vi "IncStepsMMAvg.vi"(0 "I/O chan for motor pulse":i32=7, 1 "wait time between scans (ms)":i32, 3 "Avg Num":i32=1, 5 "number of scans":i32=128, 9 "Axis":i32=1 min=1 max=4, 11 "Steps to move":i32=100, 13 "Crate File Names":string[](array[string]), 14 "Reverse ?":bool) -> ()   [LabVIEW 2022 SP3]
uses:
  <instrlib>/Acqiris Dx/Acqiris Dx.lvlib
  -MotionRoutines/MotionGlobals.vi
  <vilib>/Analysis/NI_AALBase.lvlib
  <vilib>/Analysis/baseanly.llb/Mean (DBL).vi
panel:
  out "Motion error":bool
  in  "Acq error in":errorcluster
  in  "Board ID":T1=1 min=1 max=32 step=1
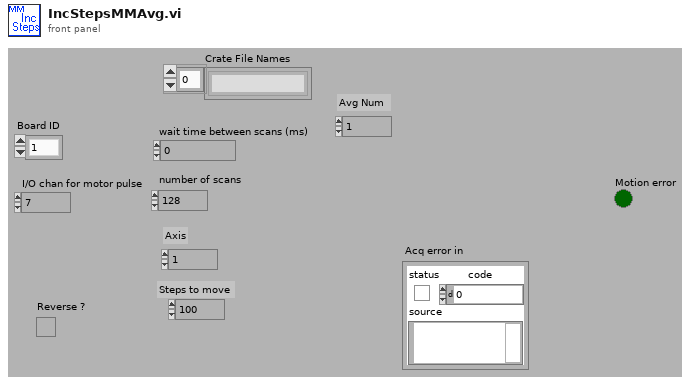
[diagram p1: front panel]
types:
  T1 = typedef "Board Id" = u8
  T2 = cluster{sgl, "Gain [dB]  ":sgl, "Atten (dB)":sgl}[]
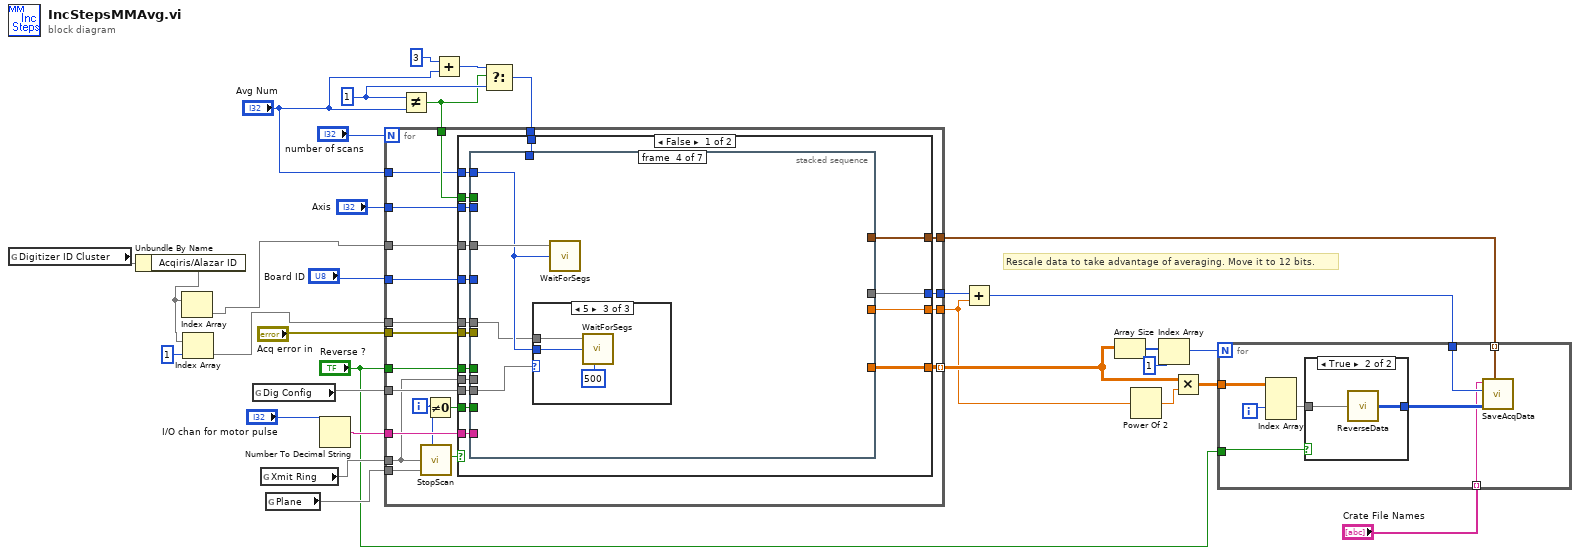
[diagram p0: block diagram]
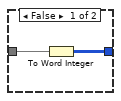
[diagram p2: hidden frame]
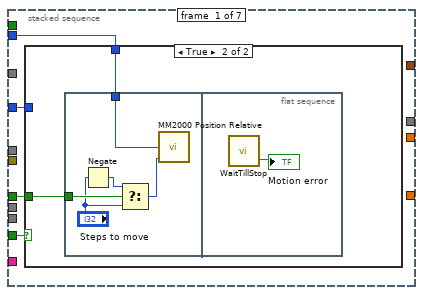
[diagram p3: hidden frame]
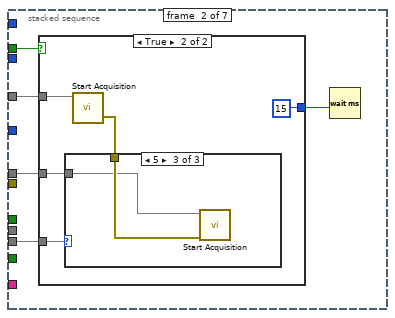
[diagram p5: hidden frame]
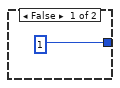
[diagram p6: hidden frame]
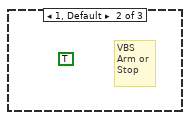
[diagram p8: hidden frame]
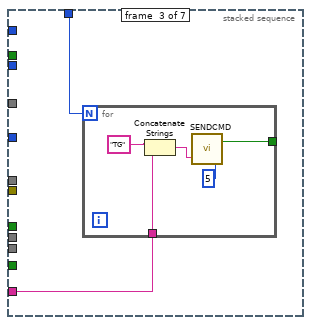
[diagram p9: hidden frame]
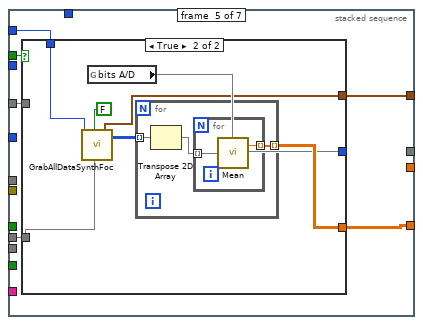
[diagram p12: hidden frame]
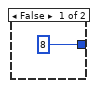
[diagram p13: hidden frame]
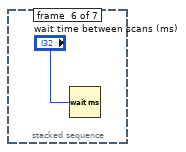
[diagram p14: hidden frame]
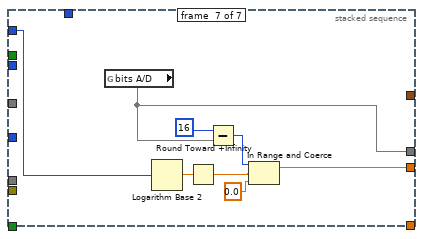
[diagram p15: hidden frame]
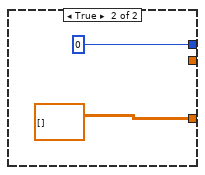
[diagram p16: hidden frame]
diagram:
  w26 = 1
  # "Rescale data to take advantage of averaging. Move it to 12 bits."
  n1 = global read "MotionGlobals.vi" "Digitizer ID Cluster"() -> (w5)
  n2 = Unbundle By Name(w5) -> ("Acqiris/Alazar ID"=w3)
  n3 = Index Array(array=w3) -> (element=w2)  [unwired: 1 in]
  n4 = Index Array(array=w3, index=1) -> (element=w1)
  n5 = global read "MotionGlobals.vi" "Dig Config"() -> (w28)
  n6 = global read "MotionGlobals.vi" "Xmit Ring"() -> (w18)
  n7 = global read "MotionGlobals.vi" "Plane"() -> (w19)
  n8 = Number To Decimal String(number="I/O chan for motor pulse") -> (decimal integer string=w21:string)  [unwired: 1 out]
  n9 = Not Equal?(x=w26, y="Avg Num") -> (x != y?=w23:bool)
  n10 = Add(x=3, y="Avg Num") -> (x+y=w24:i32)
  n11 = Select(t=w24, s=w23, f=w26) -> (s? t:f=w27:i32)
  n12 = for {
    N: "number of scans" -> [_]
    tunnel: "Board ID" -> [w52]
    tunnel: "Axis" -> [w51]
    tunnel: "Reverse ?" -> [w50]
    tunnel: w27 -> [w49]
    tunnel: w2 -> [w48]
    tunnel: "Acq error in" -> [w47]
    tunnel: w28 -> [w46]
    tunnel: [w42] -> w12 mode=indexing
    tunnel: w23 -> [w45]
    tunnel: [w43] -> w8
    tunnel: w21 -> [w40]
    tunnel: "Avg Num" -> [w39]
    tunnel: w19 -> [w37]
    tunnel: w18 -> [w36]
    tunnel: [w35] -> w9
    tunnel: [w34] -> w6
    tunnel: w1 -> [w33]
    i -> [w38]
    n13 = call "StopScan.vi"("Ring"=w36, "Current Plane"=w37, "Line Number"=w38) -> ("Stop Now? Dup"=w41:bool)  [unwired: 1 in, 2 out]
    n14 = Not Equal To 0?(x=w38) -> (x != 0?=w44:bool)
    n15 = case shown="False" w41 {
      tunnel: w52 -> [w69 _]
      tunnel: w51 -> [w68 _]
      tunnel: w50 -> [w67 _]
      tunnel: w49 -> [w66 _]
      tunnel: w48 -> [w65 _]
      tunnel: w47 -> [w64 _]
      tunnel: w46 -> [w63 _]
      tunnel: w45 -> [w62 _]
      tunnel: w44 -> [w61 _]
      tunnel: [w54 u16 0] -> w43
      tunnel: [w60 dbl[][] [] ("Data")] -> w42
      tunnel: w40 -> [w59 _]
      tunnel: w39 -> [w58 _]
      tunnel: w36 -> [w57 _]
      tunnel: [w56 _] -> w35
      tunnel: [w55 _] -> w34
      tunnel: w33 -> [w53 _]
      frame False {
        n16 = stacked-sequence {
          tunnel: w69 -> [w73 _ _ _ _ _ _]
          tunnel: w68 -> [w72 _ _ _ _ _ _]
          tunnel: w67 -> [w71 _ _ _ _ _ _]
          tunnel: w66 -> [_ _ w96 _ _ _ _]
          tunnel: w65 -> [_ w86 _ w105 w114 _ _]
          tunnel: w64 -> [_ _ _ _ _ _ _]
          tunnel: w63 -> [_ w83 _ w104 _ _ _]
          tunnel: [_ _ _ _ w110 _ _] -> w60
          tunnel: w62 -> [_ w85 _ _ w113 _ _]
          tunnel: w61 -> [w70 _ _ _ _ _ _]
          tunnel: w59 -> [_ _ w95 _ _ _ _]
          tunnel: w58 -> [_ _ _ w103 w112 _ w131]
          tunnel: w57 -> [_ _ _ _ w111 _ _]
          tunnel: [_ _ _ _ w109 _ _] -> w56
          tunnel: [_ _ _ _ _ _ w130] -> w55
          tunnel: [_ _ _ _ _ _ w129] -> w54
          tunnel: w53 -> [_ w82 _ w102 _ _ _]
          frame #0 {
            n17 = case shown="True" w70 {
              tunnel: w73 -> [_ _]
              tunnel: w72 -> [_ w74]
              tunnel: w71 -> [_ w75]
              frame False {
              }
              frame True {
                n18 = flat-sequence {
                  tunnel: w75 -> [w80]
                  tunnel: w74 -> [w77]
                  frame #0 {
                    n19 = Negate(x="Steps to move") -> (-x=w78:i32)
                    n20 = Select(t=w78, s=w80, f="Steps to move") -> (s? t:f=w76:i32)
                    n21 = call "MM2000 Position Relative.vi"("Position Relative"=w76, "Axis"=w77) -> ()  [unwired: 1 in]
                  }
                  frame #1 {
                    n22 = call "WaitTillStop.vi"() -> ("Error Status"=→"Motion error":bool)  [unwired: 3 out]
                  }
                }
              }
            }
          }
          frame #1 {
            n23 = case shown="True" w85 {
              tunnel: w86 -> [_ w92]
              tunnel: [1 15] -> w84
              tunnel: w83 -> [_ w90]
              tunnel: w82 -> [_ w88]
              frame False {
              }
              frame True {
                n24 = call <instrlib>:"Start Acquisition.vi"("Instrument ID"=w92) -> ("error out"=w89:errorcluster)  [unwired: 3 in, 1 out]
                n25 = case shown="5" w90 {
                  tunnel: w89 -> [_ _ w94]
                  tunnel: w88 -> [_ _ w93]
                  frame 0 {
                  }
                  frame 1, Default {
                    (unwired) TRUE
                    # "VBS\nArm or\nStop"
                  }
                  frame 5 {
                    n26 = call <instrlib>:"Start Acquisition.vi"("error in (no error)"=w94, "Instrument ID"=w93) -> ()  [unwired: 2 in, 2 out]
                  }
                }
              }
            }
            n27 = Wait (ms)(milliseconds to wait=w84) -> ()  [unwired: 1 out]
          }
          frame #2 {
            n28 = for {
              N: w96 -> [_]
              tunnel: [w100] -> _
              tunnel: w95 -> [w97]
              n29 = Concatenate Strings("TG", w97) -> (w98:string)
              n30 = call "SENDCMD.VI"("Wait time (ms)"=5, "MM2000 Command (ASCII String)"=w98) -> ("Boolean"=w100:bool)  [unwired: 1 in]
            }
          }
          frame #3 {
            n31 = case shown="5" w104 {
              tunnel: w102 -> [_ _ w108]
              tunnel: w103 -> [_ _ w106]
              frame 0 {
              }
              frame 1, Default {
              }
              frame 5 {
                n32 = call "WaitForSegs.vi"("Acqiris ID"=w108, "lines per plane"=w106, "Timeout"=500) -> ()  [unwired: 1 in, 4 out]
              }
            }
            n33 = call "WaitForSegs.vi"("Acqiris ID"=w105, "lines per plane"=w103) -> ()  [unwired: 2 in, 4 out]
          }
          frame #4 {
            n34 = case shown="True" w113 {
              tunnel: w114 -> [_ _]
              tunnel: [8 ("mean") w117] -> _
              tunnel: w112 -> [_ w119]
              tunnel: w111 -> [_ w118]
              tunnel: [_ w120] -> w110
              tunnel: [_ w116] -> w109
              frame False {
              }
              frame True {
                n35 = call "GrabAllDataSynthFoc.vi"("lines per plane mod"=w119, "save?"=FALSE, "Xmit Ring"=w118) -> ("Gain Array"=w116:T2, "Raw data out"=w121:i16[][][])  [unwired: 5 in, 10 out]
                n36 = global read "MotionGlobals.vi" "bits A/D"() -> (w117)
                n37 = for {
                  tunnel: w121 -> [w125] mode=indexing
                  tunnel: [w123] -> w120 mode=indexing
                  n38 = Transpose 2D Array(2D array=w125) -> (transposed array=w124:i16[][])
                  n39 = for {
                    tunnel: w124 -> [w127] mode=indexing
                    tunnel: [w126] -> w123 mode=indexing
                    n40 = call-poly <vilib>:"Mean.vi"("X"=w127) -> ("mean"=w126:dbl)  [unwired: 1 out]
                  }
                }
              }
            }
          }
          frame #5 {
            n41 = Wait (ms)(milliseconds to wait="wait time between scans (ms)") -> ()  [unwired: 1 out]
          }
          frame #6 {
            n42 = global read "MotionGlobals.vi" "bits A/D"() -> (w129)
            n43 = Logarithm Base 2(1:w131) -> (0:w136:dbl)
            n44 = Round Toward +Infinity(x=w136) -> (ceil(x): smallest int >= x=w135:dbl)
            n45 = Subtract(x=16, y=w129) -> (x-y=w132:i32)
            n46 = In Range and Coerce(upper limit=w132, x=w135, lower limit=0.0) -> (coerced(x)=w130:dbl)  [unwired: 1 out]
          }
        }
      }
      frame True {
      }
    }
  }
  n47 = Add(x=w8, y=w6) -> (x+y=w7:u16)
  n48 = Array Size(array=w12) -> (size(s)=w17:i32[])
  n49 = Power Of 2(x=w6) -> (2^x=w14:dbl)
  n50 = Index Array(array=w17, index=1) -> (element=w15:i32)
  n51 = Multiply(x=w12, y=w14) -> (x*y=w13:dbl[][][])
  n52 = for {
    N: w15 -> [_]
    tunnel: w13 -> [w146]
    tunnel: "Reverse ?" -> [w144]
    tunnel: w7 -> [w143]
    tunnel: "Crate File Names" -> [w140] mode=indexing
    tunnel: w9 -> [w139] mode=indexing
    i -> [w145]
    n53 = Index Array(array=w146, index (dim 1)=w145) -> (element=w141:dbl[][])  [unwired: 2 in]
    n54 = case shown="True" w144 {
      tunnel: w141 -> [w148 w150]
      tunnel: [w147 w149] -> w142
      frame False {
        n55 = To Word Integer(number=w148) -> (16bit integer=w147:i16[][])
      }
      frame True {
        n56 = call "ReverseData.vi"("Array in"=w150) -> ("Array out"=w149:i16[][])
      }
    }
    n57 = call "SaveAcqData.vi"("Votage scaling"=w139, "Array"=w142, "Dig Word Size"=w143, "File Name"=w140) -> ()  [unwired: 3 in]
  }
